vi "Exponential Fit.vi"(8 "Voltage (Value)":dbl, 9 "Voltage (Array)":dbl[](array[numeric]), 10 "Reference (Value)":dbl, 11 "Reference (Array)":dbl[](array[numeric])) -> (0 "Best Logarithmic Fit":dbl[](array[numeric]), 1 "Apmlitude":dbl, 2 "Voltage Out":dbl[](array[numeric]), 3 "Reference Out":dbl[](array[numeric]), 5 "scale":dbl)   [LabVIEW 2013]
uses:
  <vilib>/Analysis/NI_AALPro.lvlib
panel:
  in  "index":i32
  out "Error Out":errorcluster
  in  "Error In":errorcluster
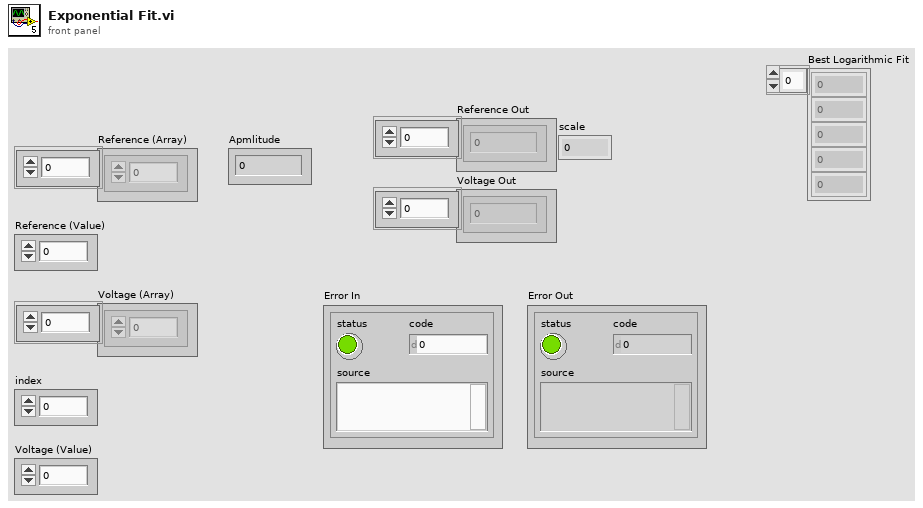
[diagram p1: front panel]
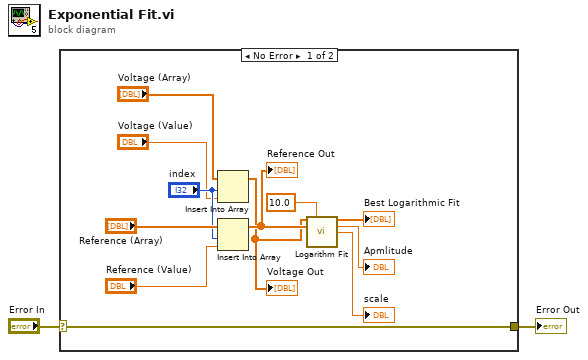
[diagram p0: block diagram]
diagram:
  n1 = case shown="No Error" "Error In" {
    selector: "Error In" -> [w9 w15]
    tunnel: [w9 w15] -> w1
    frame No Error {
      w7 = 10.0 items=["e"=2.71828, "2"=2.0, "10"=10.0] ("base")
      n2 = Insert Into Array(array="Voltage (Array)", index="index", new element="Voltage (Value)") -> (w3:dbl[])
      "Voltage Out" <- w3
      n3 = Insert Into Array(array="Reference (Array)", index="index", new element="Reference (Value)") -> (w4:dbl[])
      "Reference Out" <- w4
      n4 = call <vilib>:"Logarithm Fit.vi"("Y"=w3, "base"=w7, "X"=w4) -> ("Best Logarithm Fit"=→"Best Logarithmic Fit":dbl[], "amplitude"=→"Apmlitude":dbl, "scale"=→"scale":dbl)  [unwired: 8 in, 2 out]
    }
    frame Error {
    }
  }
  "Error Out" <- w1
